vi "Shutdown.vi"(8 "Error In":errorcluster) -> (0 "Error Out":errorcluster)   [LabVIEW 2025, in "LOGlib_LV2025.lvlib"]
doc: "Writes all remaining log statements to the default log file if enabled and properly closes all files and releases all listeners."
uses:
  LOGlib_LV2025.lvlib
  Support/File/Action.ctl
  Support/Error/Action.ctl
  Support/Action.ctl
  Support/File/File.lvlib
  Support/Error/Error.lvlib
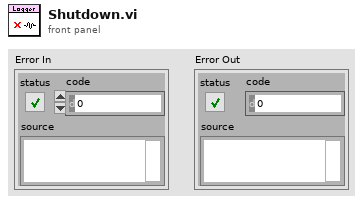
[diagram p1: front panel]
types:
  T1 = typedef "LOGlib_LV2025.lvlib/File.lvlib/Action.ctl" = enum16{"Initialize", "Set Maximum File Size", "Set Maximum File Count", "Set Root Folder", "Set Enable Calendar Folder Tree", "Set File Extension", "Set Prune All", "Set Delimiter", "Start", "Write", "Stop", "Shutdown"}
  T2 = typedef "LOGlib_LV2025.lvlib/Error.lvlib/Action.ctl" = enum16{"Initialize", "Get", "Set Verbosity", "Set User-Defined Codes", "Set User-Defined Descriptions", "Shutdown"}
  T3 = typedef "LOGlib_LV2025.lvlib/Action.ctl" = enum16{"Initialize", "Register", "Log", "Unregister", "Set Level", "Shutdown"}
  T4 = typedef "LOGlib_LV2025.lvlib/Statement.ctl" = cluster{"Time Stamp":timestamp, "Tag":T5, "Source":string, "Message":string}
  T5 = typedef "LOGlib_LV2025.lvlib/Tag.ctl" = enum16{"Fatal", "Error", "Warn", "Info", "Debug", "Trace"}
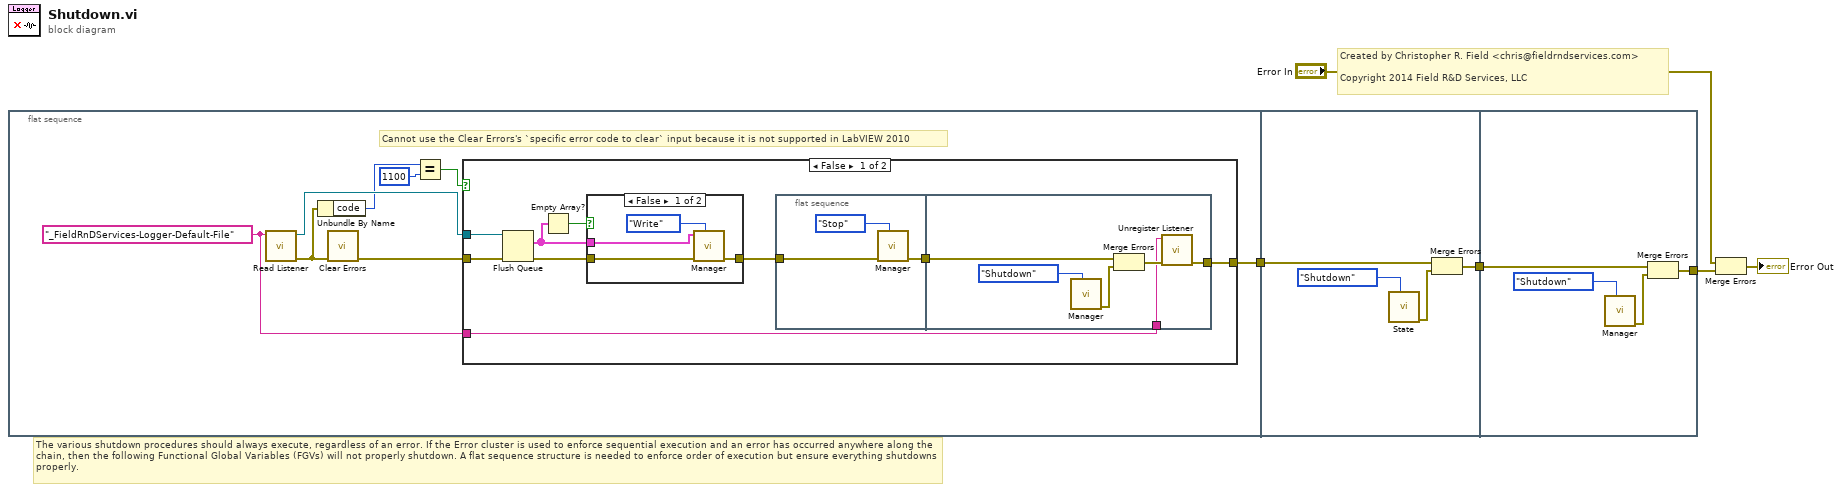
[diagram p0: block diagram]
diagram:
  # "The various shutdown procedures should always execute, regardless of an error. If the Error cluster is used to enforce sequential execution and an error has occurred anywhere along the chain, then the following Functional Global Variables (FGVs) will not properly shutdown. A flat sequence structure is needed to enforce order of execution but ensure everything shutdowns properly."
  # "Created by Christopher R. Field <chris@fieldrndservices.com>\n\nCopyright 2014 Field R&D Services, LLC"
  n1 = flat-sequence {
    tunnel: [w10] -> w1
    tunnel: [w39] -> w5
    tunnel: w1 -> [w38]
    tunnel: w5 -> [w44]
    tunnel: [w42] -> w4
    frame #0 {
      w11 = "_FieldRnDServices-Logger-Default-File" ("Listener ID")
      # "Cannot use the Clear Errors's `specific error code to clear` input because it is not supported in LabVIEW 2010"
      n2 = call "Read Listener.vi"("Listener ID"=w11) -> ("Error Out"=w9:errorcluster, "Listener"=w13:refnum<queue>)  [unwired: 9 in]
      n3 = Unbundle By Name(w9) -> ("code"=w8:i32)
      n4 = call <vilib>:"Clear Errors.vi"("error in (no error)"=w9) -> ("error out"=w12:errorcluster)  [unwired: 5 in, 1 out]
      n5 = Equal?(x=w8, y=1100 ("specific error code to clear (0: all)")) -> (x = y?=w6:bool)
      n6 = case shown="False" w6 {
        tunnel: w13 -> [w22 _]
        tunnel: w12 -> [w21 w37]
        tunnel: [w17 w37] -> w10
        tunnel: w11 -> [w16 _]
        frame False {
          n7 = Flush Queue(queue=w22, error in (no error)=w21) -> (remaining elements=w15:T4[], error out=w20:errorcluster)  [unwired: 1 out]
          n8 = Empty Array?(array=w15) -> (empty?=w14:bool)
          n9 = case shown="False" w14 {
            tunnel: w20 -> [w25 w27]
            tunnel: [w24 w27] -> w19
            tunnel: w15 -> [w23 _]
            frame False {
              n10 = call "Manager.vi"("Action"=Action."Write", "Error In"=w25, "Set Value"=w23) -> ("Error Out"=w24:errorcluster)  [unwired: 8 in]
            }
            frame True {
            }
          }
          n11 = flat-sequence {
            tunnel: w19 -> [w29]
            tunnel: [w28] -> w18
            tunnel: w18 -> [w34]
            tunnel: [w32] -> w17
            tunnel: w16 -> [w31]
            frame #0 {
              n12 = call "Manager.vi"("Action"=Action."Stop", "Error In"=w29) -> ("Error Out"=w28:errorcluster)  [unwired: 9 in]
            }
            frame #1 {
              n13 = call "Manager.vi"("Action"=Action."Shutdown") -> ("Error Out"=w36:errorcluster)  [unwired: 10 in]
              n14 = Merge Errors(w34, w36) -> (w33:errorcluster)
              n15 = call "Unregister Listener.vi"("Error In"=w33, "Listener ID"=w31) -> ("Error Out"=w32:errorcluster)  [unwired: 9 in]
            }
          }
        }
        frame True {
        }
      }
    }
    frame #1 {
      n16 = call "State.vi"("Action"=Action."Shutdown") -> ("Error Out"=w40:errorcluster)  [unwired: 9 in, 1 out]
      n17 = Merge Errors(w38, w40) -> (w39:errorcluster)
    }
    frame #2 {
      n18 = call "Manager.vi"("Action"=Action."Shutdown") -> ("Error Out"=w43:errorcluster)  [unwired: 10 in]
      n19 = Merge Errors(w44, w43) -> (w42:errorcluster)
    }
  }
  n20 = Merge Errors("Error In", w4) -> (→"Error Out":errorcluster)
